vi "Auton Turn to disired angle.vi"(7 "Power output range":cluster{"output high":dbl, "output low":dbl}={"output high"=0.4, "output low"=-0.4} {"output low" format="%.2f"; "output high" format="%.2f"}, 10 "PID Turn  gains":T1={"proportional gain (Kc)"=0.05, "integral time (Ti, min)"=0.01, "derivative time (Td, min)"=0.0} {"derivative time (Td, min)" format="%.3f"; "integral time (Ti, min)" format="%.3f"; "proportional gain (Kc)" format="%.3f"}, 11 "Angle setpoint":dbl format="%.2f") -> (3 "In Range?":bool)   [LabVIEW 2014]
uses:
  DriveGlobal.vi
  <vilib>/addons/control/pid/pid.llb/PID (DBL).vi
  Robot Values.vi
  <vilib>/addons/control/pid/NI_PID_pid.lvlib
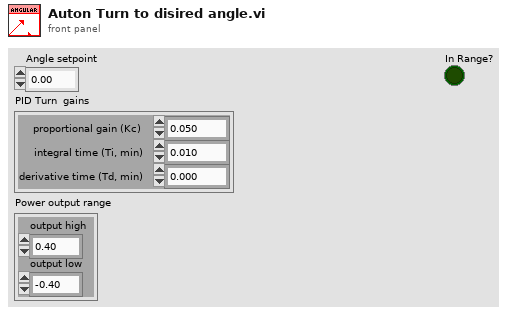
[diagram p1: front panel]
types:
  T1 = cluster{"proportional gain (Kc)":dbl, "integral time (Ti, min)":dbl, "derivative time (Td, min)":dbl}
  T2 = cluster{"Lift Encoder Height Right (cm)":dbl, "Lift Encoder Height Left (cm)":dbl, "Right Prox":bool, "Left Prox":bool, "Gyro Angle":dbl, "Gyro anglar rate":dbl, "Gyro Reset":bool}
  T3 = cluster{"RightMotorSpeed":dbl, "LeftMotorSpeed":dbl}
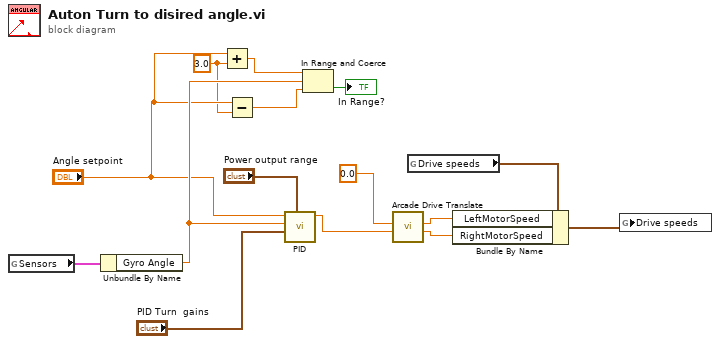
[diagram p0: block diagram]
diagram:
  w4 = 3.0 ("y")
  n1 = global read "Robot Values.vi" "Sensors"() -> (w15:T2)
  n2 = Unbundle By Name(w15) -> ("Gyro Angle"=w6:dbl)
  n3 = Add(x="Angle setpoint", y=w4) -> (x+y=w2:dbl)
  n4 = Subtract(x="Angle setpoint", y=w4) -> (x-y=w3:dbl)
  n5 = call-poly <vilib>:"PID.vi"("output range"="Power output range", "PID gains"="PID Turn  gains", "process variable"=w6, "setpoint"="Angle setpoint") -> ("output"=w11:dbl)  [unwired: 6 in, 1 out]
  n6 = In Range and Coerce(upper limit=w2, x=w6, lower limit=w3) -> (In Range?=→"In Range?":bool)  [unwired: 1 out]
  n7 = call "Arcade Drive Translate.vi"("xAxis"=w11, "yAxis"=0.0) -> ("outputX"=w7:dbl, "outputY"=w8:dbl)  [unwired: 7 in]
  n8 = global read "DriveGlobal.vi" "Drive speeds"() -> (w9:T3)
  n9 = Bundle By Name(cluster=w9, "LeftMotorSpeed"=w8, "RightMotorSpeed"=w7) -> (w10:T3)
  n10 = global write "DriveGlobal.vi" "Drive speeds"(w10) -> ()
